vi "Distance.vi"(10 "To":T1, 11 "From":T1) -> (3 "Distance":dbl)   [LabVIEW 2020, in "SquareBattle.lvlib"]
uses:
  SquareBattle.lvlib
  Position.ctl
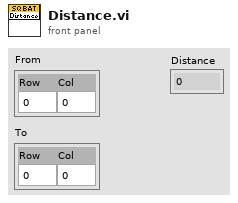
[diagram p1: front panel]
types:
  T1 = typedef "SquareBattle.lvlib/Position.ctl" = cluster{"Row":i32, "Col":i32}
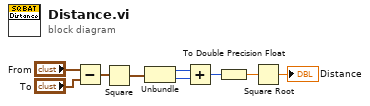
[diagram p0: block diagram]
diagram:
  n1 = Subtract(x="From", y="To") -> (x-y=w7:T1)
  n2 = Square(x=w7) -> (x^2=w6:T1)
  n3 = Unbundle(w6) -> ("Row"=w5:i32, "Col"=w4:i32)
  n4 = Add(x=w5, y=w4) -> (x+y=w3:i32)
  n5 = To Double Precision Float(number=w3) -> (double precision float=w2:dbl)
  n6 = Square Root(x=w2) -> (sqrt(x)=→"Distance":dbl)
